vi "Convert Segments.vi"(11 "Pattern String":string) -> (2 "Segment Indices":cluster{i32[]}[](array[cluster]), 3 "Length Grouped Segments":cluster{cluster{i32[]}[]}[](array[cluster]))   [LabVIEW 2020]
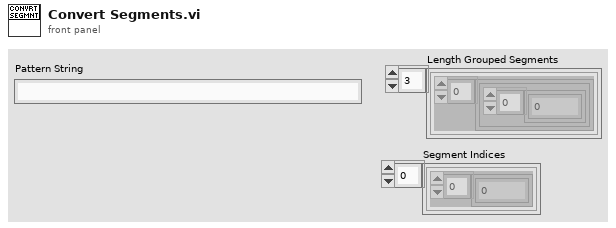
[diagram p1: front panel]
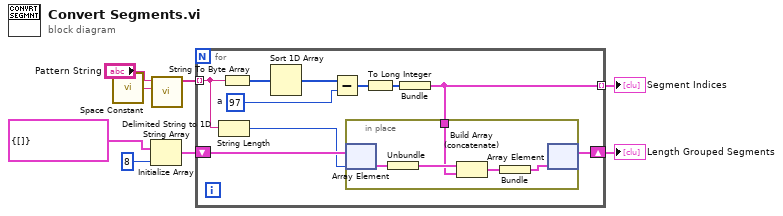
[diagram p0: block diagram]
diagram:
  n1 = call <vilib>:"Space Constant.vi"() -> ("String"=w8:string)
  n2 = Initialize Array(cluster{cluster{i32[]}[]} {[]}, 8 ("dimension size")) -> (w4:cluster{cluster{i32[]}[]}[])
  n3 = call <vilib>:"Delimited String to 1D String Array.vi"("delimiter"=w8, "delimited string"="Pattern String") -> ("string array"=w6:string[])  [unwired: 9 in]
  n4 = for {
    tunnel: w6 -> [w16] mode=indexing
    shift-right: [w12] -> w2
    shift-left: w4 -> [w15]
    tunnel: [w11] -> w1 mode=indexing
    w18 = u8 97  # a
    n5 = String Length(string=w16) -> (length=w14:i32)
    n6 = String To Byte Array(string=w16) -> (unsigned byte array=w10:u8[])
    n7 = Sort 1D Array(array=w10) -> (sorted array=w9:u8[])
    n8 = Subtract(x=w9, y=w18) -> (x-y=w17:u8[])
    n9 = To Long Integer(number=w17) -> (32bit integer=w13:i32[])
    n10 = Bundle(w13) -> (w11:cluster{i32[]})  [unwired: 1 in]
    n11 = in-place {
      in-place-border: w11 -> [w20]
      n12 = in-place-array #1(w15, w14) -> (w23:cluster{cluster{i32[]}[]})
      n13 = Unbundle(w23) -> (w22:cluster{i32[]}[])
      n14 = Build Array (concatenate)(w22, w20) -> (w21:cluster{i32[]}[])
      n15 = Bundle(w21) -> (w19:cluster{cluster{i32[]}[]})  [unwired: 1 in]
      n16 = in-place-array #1(w19) -> (w12:cluster{cluster{i32[]}[]}[])  [unwired: 1 out]
    }
  }
  "Length Grouped Segments" <- w2
  "Segment Indices" <- w1
